vi "Load_from_Project.vi"(8 "error in (no error)":errorcluster, 9 "index":i32, 10 "buildObject":T3, 11 "AB_Source_VI in":refnum<class "AB_Source_VI.lvclass">) -> (0 "error out":errorcluster, 2 "linker info":T2, 3 "AB_Source_VI out":refnum<class "AB_Source_VI.lvclass">)   [LabVIEW 2020, in "AB_Source_VI.lvclass"]
uses:
  <vilib>/AppBuilder/AB_Classes/Source/VI/AB_Source_VI.lvclass
  <resource>/Framework/Providers/API/ItemRef.ctl
  <vilib>/Utility/lvfile.llb/LVFileType.ctl
  <vilib>/AppBuilder/RW_Project/AB_RW_Project_PropBag_Action.ctl
  <vilib>/AppBuilder/AB_Classes/Source/VI/AB_Source_VI.lvclass/AB_Source_VI.ctl
  <vilib>/AppBuilder/AB_Classes/Source/AB_Source.lvclass
  <vilib>/Utility/lvfile.llb/NI_FileType.lvlib
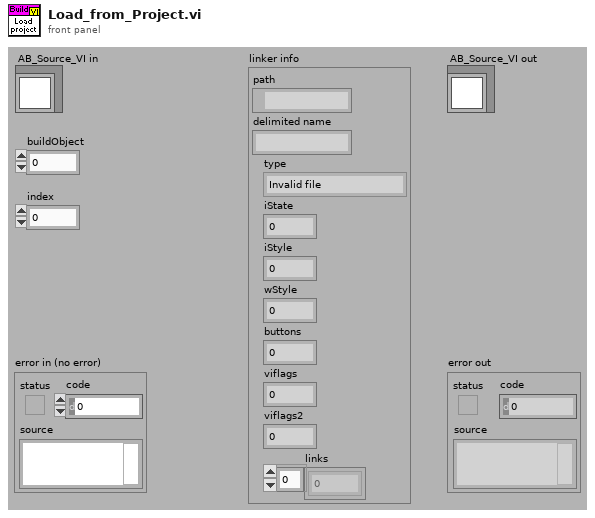
[diagram p1: front panel]
types:
  T1 = typedef "NI_FileType.lvlib/LVFileType.ctl" = enum32{"Invalid file", "Unknown type", "Instrument", "Control", "Polymorphic VI", "Project", "Library", "LVClass", "XControl", "XNode", "Shared library", ".NET assembly", "ActiveX interface", "CIN", "Run-time menu", "Palette menu", "Help file", "LLB", "XNode Edit Dependency", "Class Private Data Control", "Statechart", "MathScript .m file", "Ladder Diagram", "LVLibp", "XNode Build Dependency"}
  T2 = cluster{"path":path, "delimited name":string, "type":T1, "iState":u32, "iStyle":u16, "wStyle":u16, "buttons":u16, "viflags":u32, "viflags2":u32, "links":u32[]}
  T3 = typedef "ItemRef.ctl" = u64
  T4 = typedef "AB_RW_Project_PropBag_Action.ctl" = enum16{"read", "write", "clear", "readPrevious", "writePrevious", "clearPrevious"}
  T5 = typedef "AB_RW_Project_Source_VI_Data.ctl" = cluster{"LLBtopLevel":bool, "privateDataControl":bool}
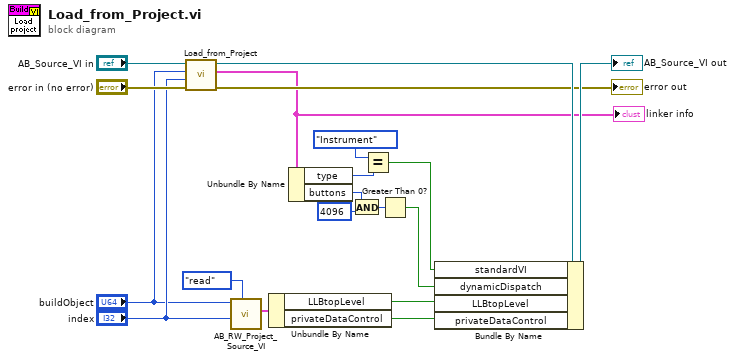
[diagram p0: block diagram]
diagram:
  n1 = call-parent "Load_from_Project.vi"("error in (no error)"="error in (no error)", "index"="index", "buildObject"="buildObject", "AB_Source in"="AB_Source_VI in") -> ("error out"=→"error out":errorcluster, "linker info"=w1:T2, "AB_Source out"=w3:refnum<class "AB_Source_VI.lvclass">)  [unwired: 5 in]
  "linker info" <- w1
  n2 = call <vilib>:"AB_RW_Project_Source_VI.vi"("action"=AB_RW_Project_PropBag_Action."read", "index in"="index", "buildObject"="buildObject") -> ("dataSource out"=w13:T5)  [unwired: 5 in, 3 out]
  n3 = Unbundle By Name(w13) -> ("LLBtopLevel"=w12:bool, "privateDataControl"=w4:bool)
  n4 = Unbundle By Name(w1) -> ("type"=w8:T1, "buttons"=w9:u16)
  n5 = And(x=w9, y=u16 4096) -> (x .and. y?=w11:u16)
  n6 = Equal?(x=LVFileType."Instrument", y=w8) -> (x = y?=w5:bool)
  n7 = Greater Than 0?(x=w11) -> (x > 0?=w6:bool)
  n8 = Bundle By Name(cluster=w3, "standardVI"=w5, "dynamicDispatch"=w6, "LLBtopLevel"=w12, "privateDataControl"=w4) -> (→"AB_Source_VI out":refnum<class "AB_Source_VI.lvclass">)
